vi "ief_set_acceleration_axis.vi"(3 "error in (no error)":errorcluster, 4 "Axis Acceleration":sgl format="%.2f", 5 "Axis Number":u16=1 min=1 max=16, 6 "Tagprefix in":refnum<k21>) -> (0 "error out (no error)":errorcluster, 1 "Axis Acceleration Out":sgl format="%.2f", 2 "Tagprefix out":refnum<k21>)   [LabVIEW 2015, in "IEF Werner.lvlib"]
doc: "The VI sets the axis acceleration of the chosen axis to the specified value. Furthermore it returns the present axis acceleration of the chosen axis after executing the set acceleration command. If the command was executed correctly the axis acceleration out is equal to the axis acceleration.\n\nAxis Number Range:\n01, 10 hex\n1, 16 dec\n\nAxis Acceleration Range: 32 Bit Float\n\nAttention:\nLeaving online mode resets the axis acceleration to values predefined by the motion control unit."
uses:
  IEF Werner.lvlib
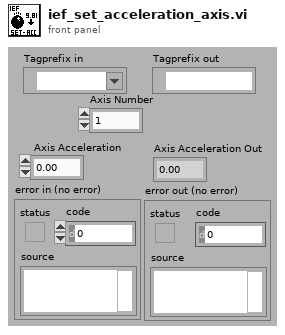
[diagram p1: front panel]
types:
  T1 = typedef "Semaphore RefNum" = refnum<k1>
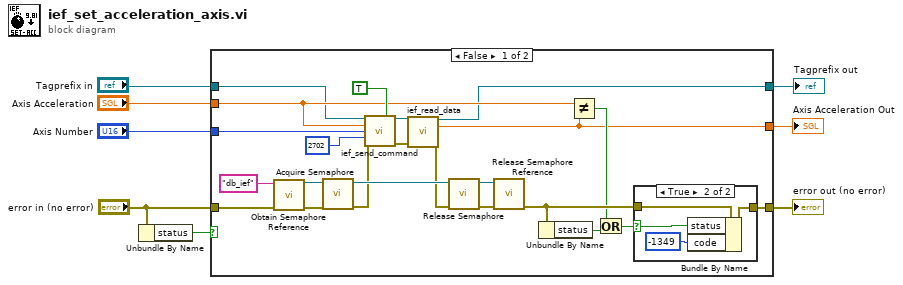
[diagram p0: block diagram]
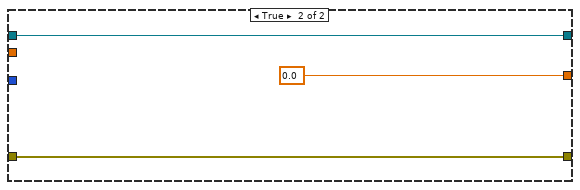
[diagram p3: hidden frame]
diagram:
  n1 = Unbundle By Name("error in (no error)") -> ("status"=w4:bool)
  n2 = case shown="False" w4 {
    tunnel: "Axis Acceleration" -> [w15 _]
    tunnel: "Axis Number" -> [w29 _]
    tunnel: "error in (no error)" -> [w20 w39]
    tunnel: [w27 w39] -> w6
    tunnel: [w12 sgl 0.0 ("value real 32")] -> w3
    tunnel: "Tagprefix in" -> [w11 w38]
    tunnel: [w9 w38] -> w1
    frame False {
      n3 = call <vilib>:"Obtain Semaphore Reference.vi"("error in (no error)"=w20, "name (unnamed)"="db_ief") -> ("error out"=w24:errorcluster, "semaphore"=w25:T1)  [unwired: 3 in, 1 out]
      n4 = call <vilib>:"Acquire Semaphore.vi"("error in (no error)"=w24, "semaphore"=w25) -> ("error out"=w19:errorcluster, "semaphore out"=w23:T1)  [unwired: 3 in, 1 out]
      n5 = call "ief_send_command.vi"("Tagprefix in"=w11, "Command datum of type real"=TRUE, "Command datum"=w15, "Command parameter"=w29, "Command code"=u16 2702, "error in (no error)"=w19) -> ("Tagprefix out"=w10:refnum<k21>, "error out (no error)"=w28:errorcluster)  [unwired: 4 in, 4 out]
      n6 = call "ief_read_data.vi"("Tagprefix in"=w10, "error in (no error)"=w28) -> ("Tagprefix out"=w9:refnum<k21>, "value real 32"=w12:sgl, "error out (no error)"=w18:errorcluster)  [unwired: 7 in, 4 out]
      n7 = call <vilib>:"Release Semaphore.vi"("error in (no error)"=w18, "semaphore"=w23) -> ("error out"=w22:errorcluster, "semaphore out"=w21:T1)  [unwired: 4 in]
      n8 = call <vilib>:"Release Semaphore Reference.vi"("error in (no error)"=w22, "semaphore"=w21) -> ("error out"=w17:errorcluster)  [unwired: 8 in, 1 out]
      n9 = Unbundle By Name(w17) -> ("status"=w13:bool)
      n10 = Not Equal?(x=w15, y=w12) -> (x != y?=w14:bool)
      n11 = Or(x=w14, y=w13) -> (x .or. y?=w16:bool)
      n12 = case shown="True" w16 {
        selector: w16 -> [_ w33]
        tunnel: [w32 w35] -> w27
        tunnel: w17 -> [w32 w36]
        frame False {
        }
        frame True {
          n13 = Bundle By Name(cluster=w36, "status"=w33, "code"=-1349) -> (w35:errorcluster)
        }
      }
    }
    frame True {
    }
  }
  "error out (no error)" <- w6
  "Axis Acceleration Out" <- w3
  "Tagprefix out" <- w1
